vi "Save Calibration Path.vi"(4 "Path":T1, 7 "Frequency":dbl[](array[numeric]), 8 "Error In":errorcluster, 9 "Measurement specfic paths":T2=enum."Harmonics", 10 "Path Loss":dbl[](array[numeric]), 11 "PathControl in":refnum<class "PathControl.lvclass">) -> (0 "Error Out":errorcluster, 3 "PathControl out":refnum<class "PathControl.lvclass">)   [LabVIEW 2020, in "PathControl.lvclass"]
uses:
  PathControl.lvclass
  Measurements Specific Paths.ctl
  Paths.ctl
  PathControl.lvclass/PathControl.ctl
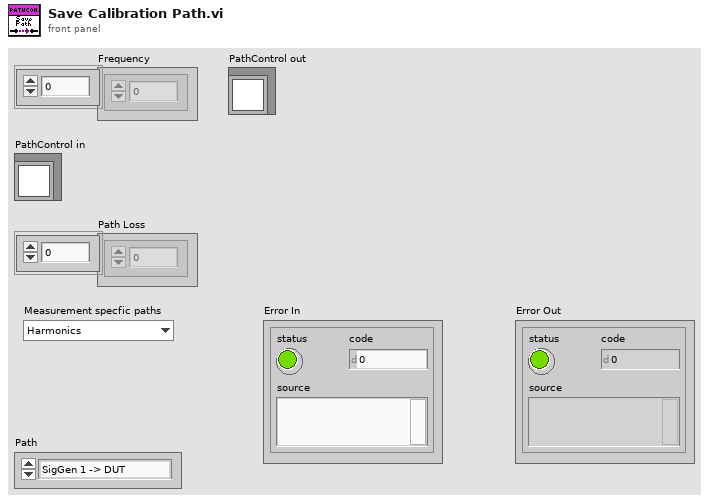
[diagram p1: front panel]
types:
  T1 = typedef "PathControl.lvclass/Paths.ctl" = enum16{"SigGen 1 -> DUT", "SigGen 2 -> DUT", "SigGen 1 -> PM 1", "SigGen 1 -> PM 2", "DUT -> SA", "DUT -> PM 2", "VSG -> DUT", "SigGen 2 -> PM 1", "SigGen 2 -> PM 2"}
  T2 = typedef "PathControl.lvclass/Measurements Specific Paths.ctl" = enum16{"No calibration", "Harmonics", "IMD", "S Parameter", "AM-AM", "MCCW-ACLR", "DC", "LCR", "Power Meter GUI", "RF Power"}
  T3 = cluster{"Name":string, "Path Frequency":dbl[], "Path Loss":dbl[]}
  T4 = cluster{"Name":string, "Path Frequency":dbl[], "Path Loss":dbl[]}[]
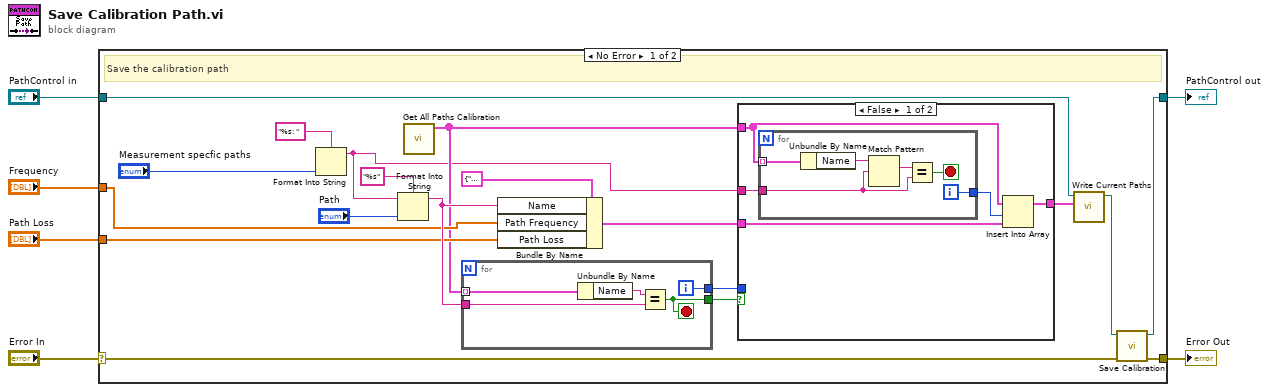
[diagram p0: block diagram]
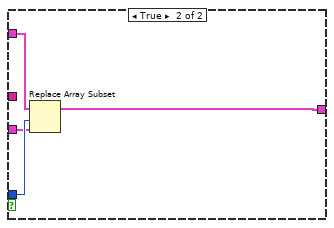
[diagram p2: hidden frame]
diagram:
  n1 = case shown="No Error" "Error In" {
    selector: "Error In" -> [w8 w46]
    tunnel: "PathControl in" -> [w14 w47]
    tunnel: "Frequency" -> [w19 _]
    tunnel: "Path Loss" -> [w18 _]
    tunnel: [w11 w47] -> w5
    tunnel: [w7 w46] -> w1
    frame No Error {
      # "Save the calibration path"
      n2 = Format Into String(format string="%s: ", "Measurement specfic paths") -> (resulting string=w9:string)  [unwired: 2 in, 1 out]
      n3 = Format Into String(format string="%s", initial string=w9, "Path") -> (resulting string=w20:string)  [unwired: 1 in, 1 out]
      n4 = call "Get All Paths Calibration.vi"() -> ("All Paths"=w17:T4)  [unwired: 10 in, 1 out]
      n5 = for {
        tunnel: w17 -> [w45] mode=indexing
        tunnel: w20 -> [w43]
        tunnel: [w42] -> w16
        tunnel: [w41] -> w10
        i -> [w42]
        stop <- w41 stop-if-true
        n6 = Unbundle By Name(w45) -> ("Name"=w44:string)
        n7 = Equal?(x=w44, y=w43) -> (x = y?=w41:bool)
      }
      n8 = Bundle By Name(cluster=T3 {"Name"="", "Path Frequency"=[], "Path Loss"=[]} ("Path"), "Name"=w20, "Path Frequency"=w19, "Path Loss"=w18) -> (w15:T3)
      n9 = case shown="False" w10 {
        tunnel: w17 -> [w26 w40]
        tunnel: w16 -> [_ w39]
        tunnel: w15 -> [w29 w38]
        tunnel: [w30 w37] -> w13
        tunnel: w9 -> [w28 _]
        frame False {
          n10 = for {
            tunnel: w26 -> [w36] mode=indexing
            tunnel: w28 -> [w33]
            tunnel: [w31] -> w27
            i -> [w31]
            stop <- w32 stop-if-true
            n11 = Unbundle By Name(w36) -> ("Name"=w35:string)
            n12 = Match Pattern(string=w35, regular expression=w33) -> (match substring=w34:string)  [unwired: 1 in, 3 out]
            n13 = Equal?(x=w34, y=w33) -> (x = y?=w32:bool)
          }
          n14 = Insert Into Array(array=w26, index=w27, new element=w29) -> (w30:T4)
        }
        frame True {
          n15 = Replace Array Subset(array=w40, new element=w38, index=w39) -> (w37:T4)
        }
      }
      n16 = call "Write Current Paths.vi"("Current Paths"=w13, "PathControl in"=w14) -> ("PathControl out"=w12:refnum<class "PathControl.lvclass">)  [unwired: 9 in]
      n17 = call "Save Calibration.vi"("error in (no error)"=w8, "PathControl in"=w12) -> ("error out"=w7:errorcluster, "PathControl out"=w11:refnum<class "PathControl.lvclass">)  [unwired: 8 in]
    }
    frame Error {
    }
  }
  "PathControl out" <- w5
  "Error Out" <- w1
